vi "Write Execute_.vi"(8 "error in (no error)":errorcluster, 10 "Execute?":bool, 11 "Read All Sensor Data Msg in":refnum<class "Read All Sensor Data Msg.lvclass">) -> (0 "error out":errorcluster, 3 "Read All Sensor Data Msg out":refnum<class "Read All Sensor Data Msg.lvclass">)   [LabVIEW 2016, in "LS218.lvlib" / "Read All Sensor Data Msg.lvclass"]
uses:
  Read All Sensor Data Msg.lvclass
  Read All Sensor Data Msg.lvclass/Read All Sensor Data Msg.ctl
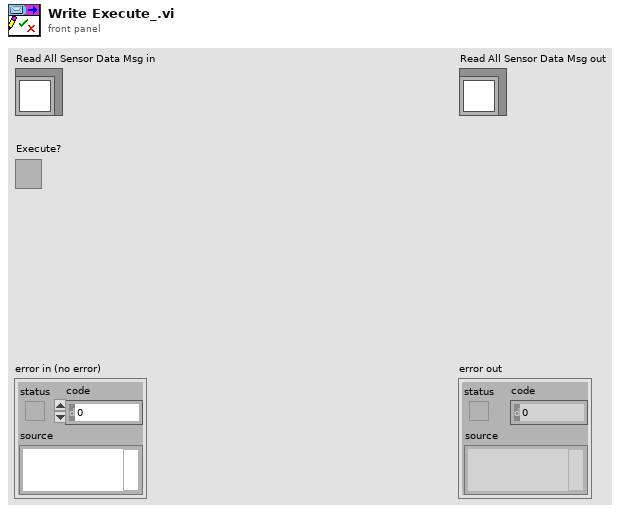
[diagram p1: front panel]
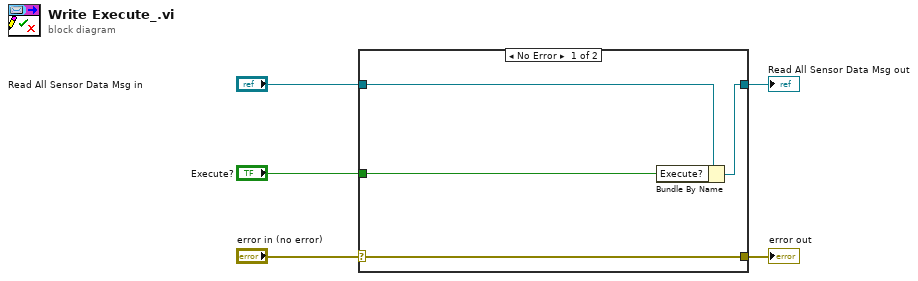
[diagram p0: block diagram]
diagram:
  n1 = case shown="No Error" "error in (no error)" {
    selector: "error in (no error)" -> [w9 w10]
    tunnel: [w9 w10] -> w4
    tunnel: [w7 w11] -> w2
    tunnel: "Read All Sensor Data Msg in" -> [w8 w11]
    tunnel: "Execute?" -> [w6 _]
    frame No Error {
      n2 = Bundle By Name(cluster=w8, "Execute?"=w6) -> (w7:refnum<class "Read All Sensor Data Msg.lvclass">)
    }
    frame Error {
    }
  }
  "error out" <- w4
  "Read All Sensor Data Msg out" <- w2
